vi "ep_Write Nominal Sampling Rate.vi"(8 "error in (no error)":errorcluster, 10 "samples per cycle":u16=9600, 11 "system info in":refnum<class "EP System Info.lvclass">) -> (0 "error out":errorcluster, 2 "nominal sampling rate [Hz]":u16, 3 "system info out":refnum<class "EP System Info.lvclass">)   [LabVIEW 2011, in "NI_EP_Power Quality.lvlib" / "EP System Info.lvclass"]
uses:
  <vilib>/addons/Electrical Power/PQ/Common/Classes/System Info/EP System Info.lvclass
  <vilib>/addons/Electrical Power/PQ/Common/Classes/System Info/EP System Info.lvclass/EP System Info.ctl
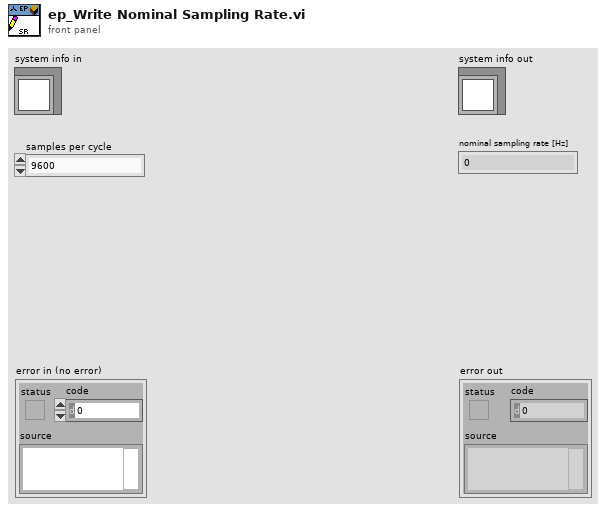
[diagram p1: front panel]
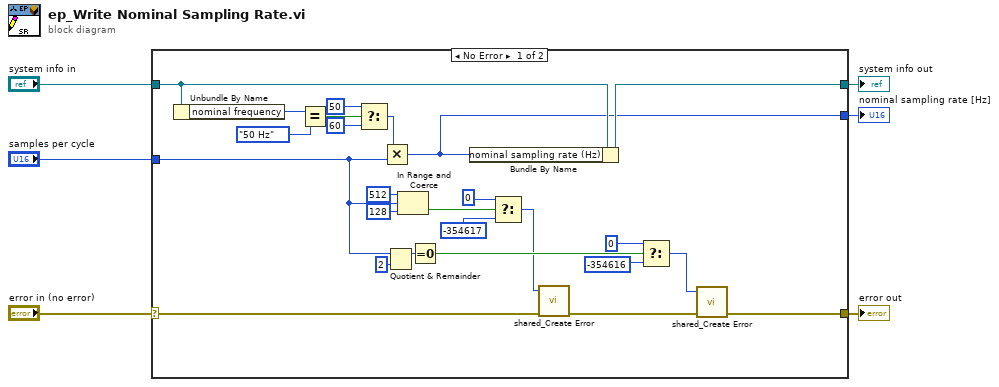
[diagram p0: block diagram]
diagram:
  n1 = case shown="No Error" "error in (no error)" {
    selector: "error in (no error)" -> [w13 w32]
    tunnel: [w8 w32] -> w5
    tunnel: [w31 w33] -> w3
    tunnel: "system info in" -> [w25 w33]
    tunnel: "samples per cycle" -> [w18 _]
    tunnel: [w16 _] -> w1
    frame No Error {
      n2 = Unbundle By Name(w25) -> ("nominal frequency"=w24:enum16{"50 Hz", "60 Hz"})
      n3 = Equal?(x=w24, y=enum16{"50 Hz", "60 Hz"}."50 Hz") -> (x = y?=w22:bool)
      n4 = Select(t=u16 50 ("y"), s=w22, f=u16 60 ("y")) -> (s? t:f=w19:u16)
      n5 = Multiply(x=w19, y=w18) -> (x*y=w16:u16)
      n6 = Quotient & Remainder(x=w18, y=u16 2) -> (x-y*floor(x/y)=w28:u16)  [unwired: 1 out]
      n7 = In Range and Coerce(upper limit=u16 512, x=w18, lower limit=u16 128) -> (In Range?=w27:bool)  [unwired: 1 out]
      n8 = Equal To 0?(x=w28) -> (x = 0?=w26:bool)
      n9 = Bundle By Name(cluster=w25, "nominal sampling rate (Hz)"=w16) -> (w31:refnum<class "EP System Info.lvclass">)
      n10 = Select(t=0 ("upper limit"), s=w27, f=-354617 ("upper limit")) -> (s? t:f=w12:i32)
      n11 = call <vilib>:"shared_Create Error.vi"("error in (no error)"=w13, "error code (0)"=w12) -> ("error out"=w10:errorcluster)  [unwired: 9 in]
      n12 = Select(t=0 ("upper limit"), s=w26, f=-354616 ("upper limit")) -> (s? t:f=w9:i32)
      n13 = call <vilib>:"shared_Create Error.vi"("error in (no error)"=w10, "error code (0)"=w9) -> ("error out"=w8:errorcluster)  [unwired: 9 in]
    }
    frame Error {
    }
  }
  "error out" <- w5
  "system info out" <- w3
  "nominal sampling rate [Hz]" <- w1
